vi "Template_GUI.vi"(11 "GUI_cluster":T1={"Sub Panel"=refnum, "GUIdevice"="Bella_LP_Mode", "CtlRef"=refnum, "User Event in"=refnum}) -> ()   [LabVIEW 2013]
uses:
  Shared/GUI_Template/GUI_master/tcp_new_data_event.ctl
  Shared/GUI_Template/GUI_master/tcp new data cluster.ctl
  Controls/GUI_cluster.ctl
  Controls/eventtypdef1.ctl
panel:
  in  "stop 2":refnum<vi>
  out "tcp data event":T2
  out "GUIdevice 1":string="Bella_LP_Mode"
  in  "stop":bool
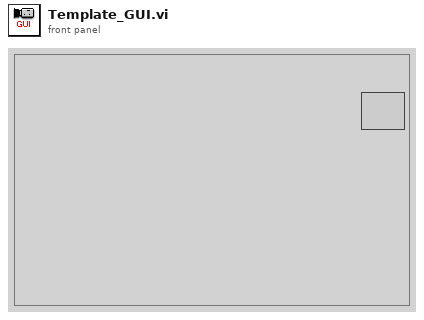
[diagram p1: front panel]
types:
  T1 = typedef "GUI_cluster.ctl" = cluster{"Sub Panel":refnum<vi>, "GUIdevice":string, "CtlRef":refnum<vi>, "User Event in":refnum<user-event>}
  T2 = typedef "tcp_new_data_event.ctl" = refnum<user-event>
  T3 = typedef "eventtypdef1.ctl" = cluster{"label":string, "Sub Panel":refnum<vi>, "CtlRef":refnum<vi>, "This VI":refnum<vi>}
  T4 = typedef "tcp new data cluster.ctl" = cluster{"EventEnum":enum16{"new data", "connection status update"}, "Device name":string}
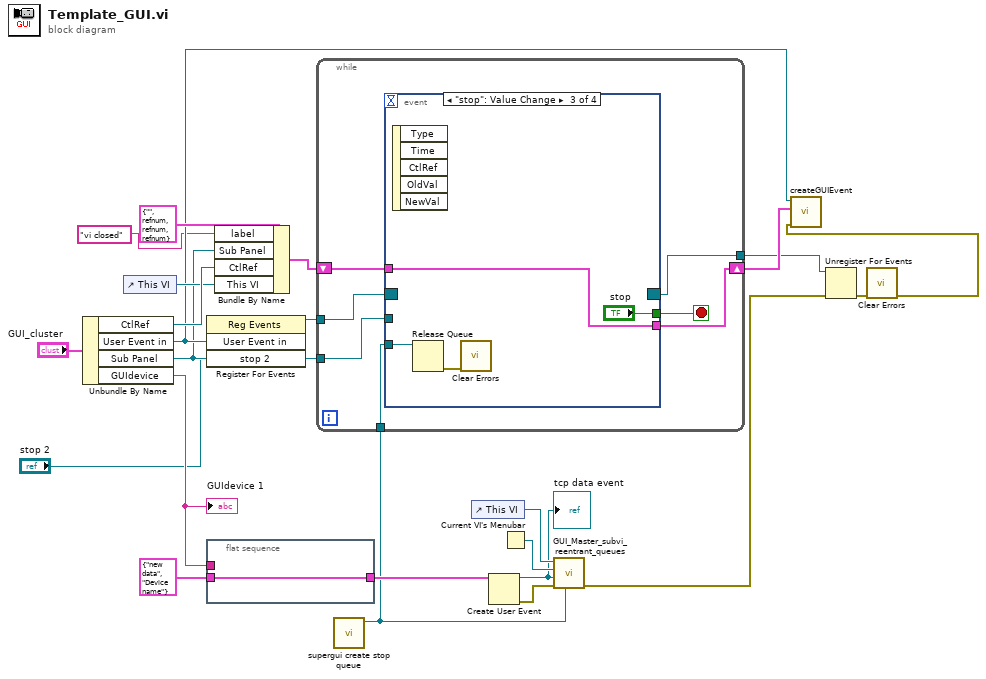
[diagram p0: block diagram]
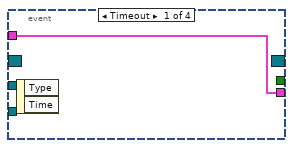
[diagram p2: hidden frame]
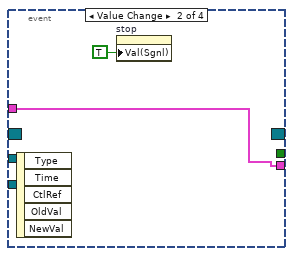
[diagram p3: hidden frame]
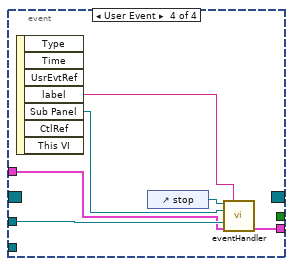
[diagram p4: hidden frame]
diagram:
  n1 = Unbundle By Name("GUI_cluster") -> ("CtlRef"=w15:refnum<vi>, "User Event in"=w11:refnum<user-event>, "Sub Panel"=w9:refnum<vi>, "GUIdevice"=w13:string)
  "GUIdevice 1" <- w13
  n2 = control-ref of="This VI"() -> (w14:refnum<vi>)
  n3 = register-events(w11, "stop 2") -> (reference out=w10:refnum<event-registration>)  [unwired: 2 in, 1 out]
  n4 = flat-sequence {
    tunnel: T4 {"EventEnum"=enum."new data", "Device name"="Device name"} ("New Event") -> [w24]
    tunnel: [w24] -> w16
    tunnel: w13 -> [_]
    frame #0 {
    }
  }
  n5 = Bundle By Name(cluster=T3 {"label"="", "Sub Panel"=refnum, "CtlRef"=refnum, "This VI"=refnum} ("event data"), "label"="vi closed", "Sub Panel"=w9, "CtlRef"=w15, "This VI"=w14) -> (w12:T3)
  n6 = call "supergui create stop queue.vi"() -> ("STOP Queue out"=w1:refnum<queue>)  [unwired: 11 in]
  n7 = while {
    shift-right: [w29] -> w8
    shift-left: w12 -> [w30]
    tunnel: w10 -> [w28]
    tunnel: w9 -> [w27]
    tunnel: [w26] -> w2
    tunnel: w1 -> [w25]
    stop <- w31 stop-if-true
    n8 = event shown="[2] \"stop\": Value Change" {
      selector: w28 -> [_ _ _ _]
      dyn-events: [_ _ _ _] -> w26
      timeout: _ -> [_ _ _ _]
      tunnel: [_ _ "stop" _] -> w31
      tunnel: w30 -> [w32 w34 w37 w41]
      tunnel: [w32 w34 w37 w40] -> w29
      tunnel: w27 -> [_ _ _ w42]
      tunnel: w25 -> [_ _ w36 _]
      event Timeout {
        n9 = event-data() -> ()  [unwired: 1 in, 2 out]
      }
      event Value Change {
        n10 = event-data() -> ()  [unwired: 1 in, 5 out]
        n11 = property on="stop" class="Bool (strict)"("Val(Sgnl)"=TRUE ("Value (Signaling)")) -> ()  [unwired: 2 in, 2 out]
      }
      event "stop": Value Change {
        n12 = event-data() -> ()  [unwired: 1 in, 5 out]
        n13 = Release Queue(queue=w36) -> (error out=w35:errorcluster)  [unwired: 2 in, 2 out]
        n14 = call <vilib>:"Clear Errors.vi"("error in (no error)"=w35) -> ()  [unwired: 6 in, 1 out]
      }
      event User Event {
        n15 = event-data() -> ("label"=w39:string, "Sub Panel"=w43:refnum<vi>)  [unwired: 1 in, 5 out]
        n16 = control-ref of="stop"() -> (w44:refnum<vi>)
        n17 = call "eventHandler.vi"("Boolean in"=w44, "label"=w39, "Sub Panel 2"=w43, "Sub Panel"=w42, "event data in"=w41) -> ("event data out"=w40:T3)  [unwired: 10 in]
      }
    }
  }
  n18 = control-ref of="This VI"() -> (w23:refnum<vi>)
  n19 = Create User Event(user event datatype=w16) -> (user event=w20:refnum<user-event>, error out=w21:errorcluster)  [unwired: 1 in]
  "tcp data event" <- w20
  n20 = Current VI's Menubar() -> (w22:refnum<k9>)
  n21 = call "GUI_Master_subvi_reentrant_queues.vi"("STOP Queue in"=w1, "error in (no error)"=w21, "tcp data event"=w20, "Caller menu reference"=w22, "Caller VI ref"=w23) -> ("error out"=w4:errorcluster)  [unwired: 6 in]
  n22 = Unregister For Events(event registration refnum=w2, error in=w4) -> (error out=w5:errorcluster)
  n23 = call <vilib>:"Clear Errors.vi"("error in (no error)"=w5) -> ("error out"=w3:errorcluster)  [unwired: 6 in]
  n24 = call "createGUIEvent.vi"("error in (no error)"=w3, "event data"=w8, "User Event in"=w11) -> ()  [unwired: 8 in, 1 out]
